vi "PXI UUT Control.vi"(1 "Enable Relays":bool, 2 "Reset IO":bool, 3 "error in (no error)":errorcluster {"code" format="%.0x"}, 4 "Enum":T2(ring), 5 "topology name":T1="2566/16-SPDT", 6 "resource name":refnum<k15>="PXI1Slot6") -> (0 "error out":errorcluster)   [LabVIEW 2014]
doc: "This VI conrtols the PXI communication streering relays.\nThe rountimes are:\n\nInit"
uses:
  <instrlib>/niSwitch/niswitch.llb/niSwitch Relay Action.ctl
  <instrlib>/niSwitch/niswitch.llb/niSwitch Topologies.ctl
panel:
  out "instrument handle out":refnum<k15>
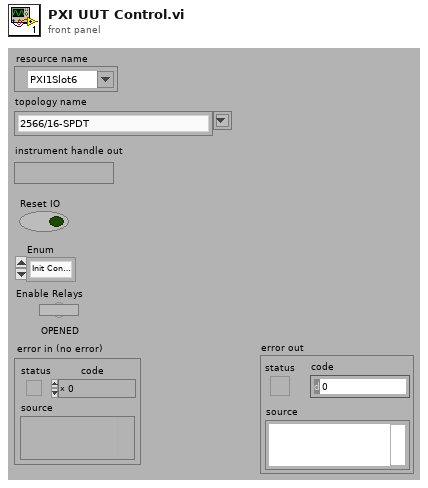
[diagram p1: front panel]
types:
  T1 = typedef "niSwitch Topologies.ctl" = string
  T2 = enum16{"Init Control Relays", "Secondary RS232", "Term Loopback", "CTS Isolate", "Synapse Loopback", "CST RTS Loopback", "Command Flash", "Auxillary RS232", "Battery Charge", "Remote Power", "Cordless Boot", "Auxillary Port", "DeInit Control Relays"}
  T3 = typedef "niSwitch Relay Action.ctl" = i32
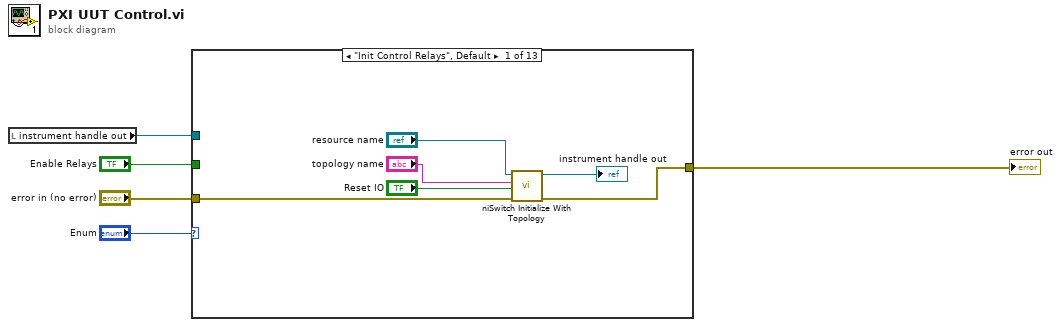
[diagram p0: block diagram]
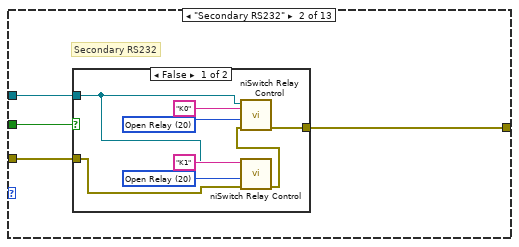
[diagram p2: hidden frame]
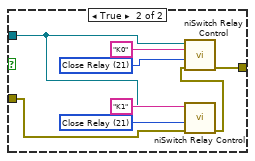
[diagram p3: hidden frame]
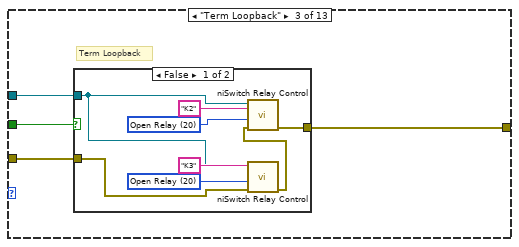
[diagram p4: hidden frame]
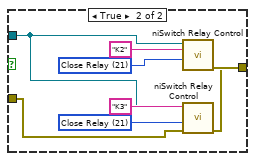
[diagram p5: hidden frame]
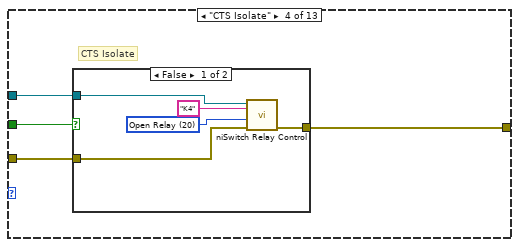
[diagram p6: hidden frame]
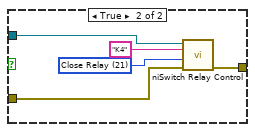
[diagram p7: hidden frame]
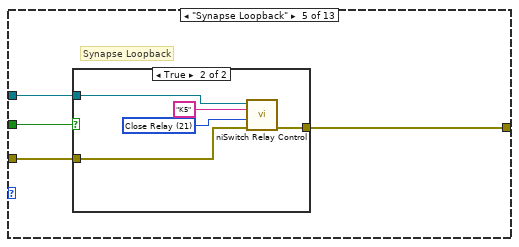
[diagram p8: hidden frame]
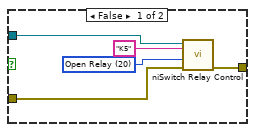
[diagram p9: hidden frame]
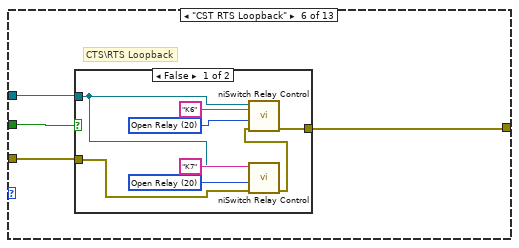
[diagram p10: hidden frame]
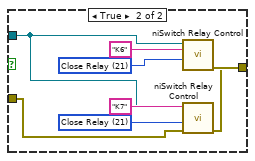
[diagram p11: hidden frame]
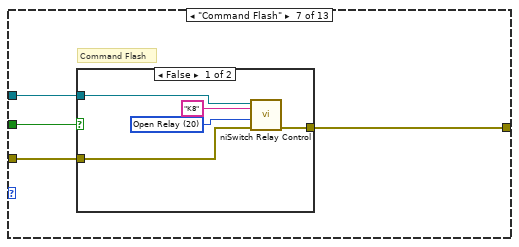
[diagram p12: hidden frame]
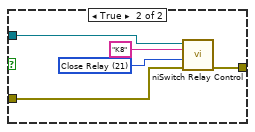
[diagram p13: hidden frame]
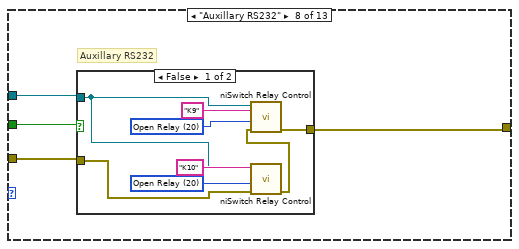
[diagram p14: hidden frame]
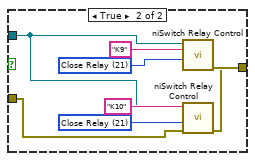
[diagram p15: hidden frame]
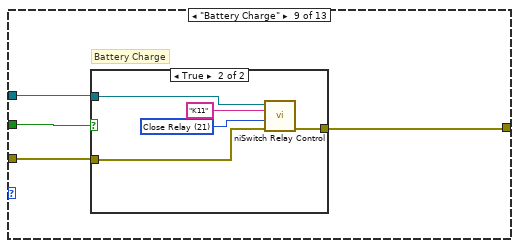
[diagram p16: hidden frame]
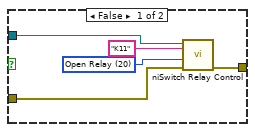
[diagram p17: hidden frame]
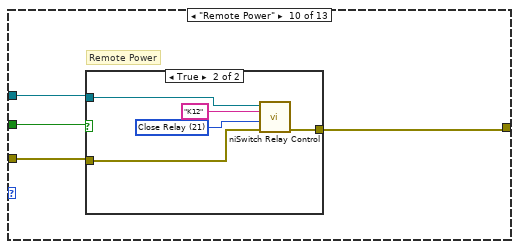
[diagram p18: hidden frame]
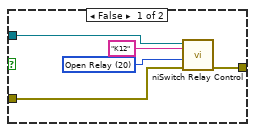
[diagram p19: hidden frame]
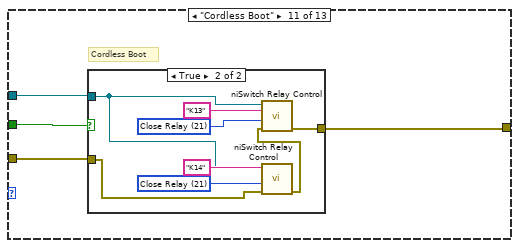
[diagram p20: hidden frame]
diagram:
  n1 = local read "instrument handle out"() -> (w4:refnum<k15>)
  n2 = case shown="\"Init Control Relays\", Default" "Enum" {
    tunnel: w4 -> [_ w15 w35 w55 w69 w83 w103 w117 w137 w151 w165 w184 w188]
    tunnel: [w11 w14 w32 w52 w66 w80 w100 w114 w134 w148 w162 w182 w185] -> w3
    tunnel: "Enable Relays" -> [_ w13 w34 w54 w68 w82 w102 w116 w136 w150 w164 _ w187]
    tunnel: "error in (no error)" -> [w10 w12 w33 w53 w67 w81 w101 w115 w135 w149 w163 w183 w186]
    frame "Init Control Relays", Default {
      n3 = call <instrlib>:"niSwitch Initialize With Topology.vi"("error in (no error)"=w10, "reset device (boolean value)"="Reset IO", "topology name"="topology name", "resource name"="resource name") -> ("error out"=w11:errorcluster, "instrument handle out"=→"instrument handle out":refnum<k15>)  [unwired: 6 in]
    }
    frame "Secondary RS232" {
      # "Secondary RS232"
      n4 = case shown="False" w13 {
        tunnel: [w21 w29] -> w14
        tunnel: w15 -> [w16 w24]
        tunnel: w12 -> [w17 w25]
        frame False {
          w20 = T3 20 items=["Open Relay"=20, "Close Relay"=21] ("relay action (Close Relay)")
          w23 = T3 20 items=["Open Relay"=20, "Close Relay"=21] ("relay action (Close Relay)")
          n5 = call <instrlib>:"niSwitch Relay Control.vi"("error in (no error)"=w17, "relay action (Close Relay)"=w20, "relay name"="K1", "instrument handle"=w16) -> ("error out"=w18:errorcluster)  [unwired: 6 in, 1 out]
          n6 = call <instrlib>:"niSwitch Relay Control.vi"("error in (no error)"=w18, "relay action (Close Relay)"=w23, "relay name"="K0", "instrument handle"=w16) -> ("error out"=w21:errorcluster)  [unwired: 6 in, 1 out]
        }
        frame True {
          w28 = T3 21 items=["Open Relay"=20, "Close Relay"=21] ("relay action (Close Relay)")
          w31 = T3 21 items=["Open Relay"=20, "Close Relay"=21] ("relay action (Close Relay)")
          n7 = call <instrlib>:"niSwitch Relay Control.vi"("error in (no error)"=w25, "relay action (Close Relay)"=w28, "relay name"="K1", "instrument handle"=w24) -> ("error out"=w26:errorcluster)  [unwired: 6 in, 1 out]
          n8 = call <instrlib>:"niSwitch Relay Control.vi"("error in (no error)"=w26, "relay action (Close Relay)"=w31, "relay name"="K0", "instrument handle"=w24) -> ("error out"=w29:errorcluster)  [unwired: 6 in, 1 out]
        }
      }
    }
    frame "Term Loopback" {
      # "Term Loopback"
      n9 = case shown="False" w34 {
        tunnel: w35 -> [w38 w46]
        tunnel: [w41 w49] -> w32
        tunnel: w33 -> [w36 w44]
        frame False {
          w40 = T3 20 items=["Open Relay"=20, "Close Relay"=21] ("relay action (Close Relay)")
          w43 = T3 20 items=["Open Relay"=20, "Close Relay"=21] ("relay action (Close Relay)")
          n10 = call <instrlib>:"niSwitch Relay Control.vi"("error in (no error)"=w36, "relay action (Close Relay)"=w40, "relay name"="K3", "instrument handle"=w38) -> ("error out"=w37:errorcluster)  [unwired: 6 in, 1 out]
          n11 = call <instrlib>:"niSwitch Relay Control.vi"("error in (no error)"=w37, "relay action (Close Relay)"=w43, "relay name"="K2", "instrument handle"=w38) -> ("error out"=w41:errorcluster)  [unwired: 6 in, 1 out]
        }
        frame True {
          w48 = T3 21 items=["Open Relay"=20, "Close Relay"=21] ("relay action (Close Relay)")
          w51 = T3 21 items=["Open Relay"=20, "Close Relay"=21] ("relay action (Close Relay)")
          n12 = call <instrlib>:"niSwitch Relay Control.vi"("error in (no error)"=w44, "relay action (Close Relay)"=w48, "relay name"="K3", "instrument handle"=w46) -> ("error out"=w45:errorcluster)  [unwired: 6 in, 1 out]
          n13 = call <instrlib>:"niSwitch Relay Control.vi"("error in (no error)"=w45, "relay action (Close Relay)"=w51, "relay name"="K2", "instrument handle"=w46) -> ("error out"=w49:errorcluster)  [unwired: 6 in, 1 out]
        }
      }
    }
    frame "CTS Isolate" {
      # "CTS Isolate"
      n14 = case shown="False" w54 {
        tunnel: w55 -> [w57 w62]
        tunnel: [w58 w63] -> w52
        tunnel: w53 -> [w56 w61]
        frame False {
          w60 = T3 20 items=["Open Relay"=20, "Close Relay"=21] ("relay action (Close Relay)")
          n15 = call <instrlib>:"niSwitch Relay Control.vi"("error in (no error)"=w56, "relay action (Close Relay)"=w60, "relay name"="K4", "instrument handle"=w57) -> ("error out"=w58:errorcluster)  [unwired: 6 in, 1 out]
        }
        frame True {
          w65 = T3 21 items=["Open Relay"=20, "Close Relay"=21] ("relay action (Close Relay)")
          n16 = call <instrlib>:"niSwitch Relay Control.vi"("error in (no error)"=w61, "relay action (Close Relay)"=w65, "relay name"="K4", "instrument handle"=w62) -> ("error out"=w63:errorcluster)  [unwired: 6 in, 1 out]
        }
      }
    }
    frame "Synapse Loopback" {
      # "Synapse Loopback"
      n17 = case shown="True" w68 {
        tunnel: w69 -> [w71 w76]
        tunnel: [w72 w77] -> w66
        tunnel: w67 -> [w70 w75]
        frame False {
          w74 = T3 20 items=["Open Relay"=20, "Close Relay"=21] ("relay action (Close Relay)")
          n18 = call <instrlib>:"niSwitch Relay Control.vi"("error in (no error)"=w70, "relay action (Close Relay)"=w74, "relay name"="K5", "instrument handle"=w71) -> ("error out"=w72:errorcluster)  [unwired: 6 in, 1 out]
        }
        frame True {
          w79 = T3 21 items=["Open Relay"=20, "Close Relay"=21] ("relay action (Close Relay)")
          n19 = call <instrlib>:"niSwitch Relay Control.vi"("error in (no error)"=w75, "relay action (Close Relay)"=w79, "relay name"="K5", "instrument handle"=w76) -> ("error out"=w77:errorcluster)  [unwired: 6 in, 1 out]
        }
      }
    }
    frame "CST RTS Loopback" {
      # "CTS\\RTS Loopback"
      n20 = case shown="False" w82 {
        tunnel: w83 -> [w86 w94]
        tunnel: [w89 w97] -> w80
        tunnel: w81 -> [w84 w92]
        frame False {
          w88 = T3 20 items=["Open Relay"=20, "Close Relay"=21] ("relay action (Close Relay)")
          w91 = T3 20 items=["Open Relay"=20, "Close Relay"=21] ("relay action (Close Relay)")
          n21 = call <instrlib>:"niSwitch Relay Control.vi"("error in (no error)"=w84, "relay action (Close Relay)"=w88, "relay name"="K7", "instrument handle"=w86) -> ("error out"=w85:errorcluster)  [unwired: 6 in, 1 out]
          n22 = call <instrlib>:"niSwitch Relay Control.vi"("error in (no error)"=w85, "relay action (Close Relay)"=w91, "relay name"="K6", "instrument handle"=w86) -> ("error out"=w89:errorcluster)  [unwired: 6 in, 1 out]
        }
        frame True {
          w96 = T3 21 items=["Open Relay"=20, "Close Relay"=21] ("relay action (Close Relay)")
          w99 = T3 21 items=["Open Relay"=20, "Close Relay"=21] ("relay action (Close Relay)")
          n23 = call <instrlib>:"niSwitch Relay Control.vi"("error in (no error)"=w92, "relay action (Close Relay)"=w96, "relay name"="K7", "instrument handle"=w94) -> ("error out"=w93:errorcluster)  [unwired: 6 in, 1 out]
          n24 = call <instrlib>:"niSwitch Relay Control.vi"("error in (no error)"=w93, "relay action (Close Relay)"=w99, "relay name"="K6", "instrument handle"=w94) -> ("error out"=w97:errorcluster)  [unwired: 6 in, 1 out]
        }
      }
    }
    frame "Command Flash" {
      # "Command Flash"
      n25 = case shown="False" w102 {
        tunnel: w103 -> [w105 w110]
        tunnel: [w106 w111] -> w100
        tunnel: w101 -> [w104 w109]
        frame False {
          w108 = T3 20 items=["Open Relay"=20, "Close Relay"=21] ("relay action (Close Relay)")
          n26 = call <instrlib>:"niSwitch Relay Control.vi"("error in (no error)"=w104, "relay action (Close Relay)"=w108, "relay name"="K8", "instrument handle"=w105) -> ("error out"=w106:errorcluster)  [unwired: 6 in, 1 out]
        }
        frame True {
          w113 = T3 21 items=["Open Relay"=20, "Close Relay"=21] ("relay action (Close Relay)")
          n27 = call <instrlib>:"niSwitch Relay Control.vi"("error in (no error)"=w109, "relay action (Close Relay)"=w113, "relay name"="K8", "instrument handle"=w110) -> ("error out"=w111:errorcluster)  [unwired: 6 in, 1 out]
        }
      }
    }
    frame "Auxillary RS232" {
      # "Auxillary RS232"
      n28 = case shown="False" w116 {
        tunnel: w117 -> [w120 w128]
        tunnel: [w123 w131] -> w114
        tunnel: w115 -> [w118 w126]
        frame False {
          w122 = T3 20 items=["Open Relay"=20, "Close Relay"=21] ("relay action (Close Relay)")
          w125 = T3 20 items=["Open Relay"=20, "Close Relay"=21] ("relay action (Close Relay)")
          n29 = call <instrlib>:"niSwitch Relay Control.vi"("error in (no error)"=w118, "relay action (Close Relay)"=w122, "relay name"="K10", "instrument handle"=w120) -> ("error out"=w119:errorcluster)  [unwired: 6 in, 1 out]
          n30 = call <instrlib>:"niSwitch Relay Control.vi"("error in (no error)"=w119, "relay action (Close Relay)"=w125, "relay name"="K9", "instrument handle"=w120) -> ("error out"=w123:errorcluster)  [unwired: 6 in, 1 out]
        }
        frame True {
          w130 = T3 21 items=["Open Relay"=20, "Close Relay"=21] ("relay action (Close Relay)")
          w133 = T3 21 items=["Open Relay"=20, "Close Relay"=21] ("relay action (Close Relay)")
          n31 = call <instrlib>:"niSwitch Relay Control.vi"("error in (no error)"=w126, "relay action (Close Relay)"=w130, "relay name"="K10", "instrument handle"=w128) -> ("error out"=w127:errorcluster)  [unwired: 6 in, 1 out]
          n32 = call <instrlib>:"niSwitch Relay Control.vi"("error in (no error)"=w127, "relay action (Close Relay)"=w133, "relay name"="K9", "instrument handle"=w128) -> ("error out"=w131:errorcluster)  [unwired: 6 in, 1 out]
        }
      }
    }
    frame "Battery Charge" {
      # "Battery Charge"
      n33 = case shown="True" w136 {
        tunnel: w137 -> [w139 w144]
        tunnel: [w140 w145] -> w134
        tunnel: w135 -> [w138 w143]
        frame False {
          w142 = T3 20 items=["Open Relay"=20, "Close Relay"=21] ("relay action (Close Relay)")
          n34 = call <instrlib>:"niSwitch Relay Control.vi"("error in (no error)"=w138, "relay action (Close Relay)"=w142, "relay name"="K11", "instrument handle"=w139) -> ("error out"=w140:errorcluster)  [unwired: 6 in, 1 out]
        }
        frame True {
          w147 = T3 21 items=["Open Relay"=20, "Close Relay"=21] ("relay action (Close Relay)")
          n35 = call <instrlib>:"niSwitch Relay Control.vi"("error in (no error)"=w143, "relay action (Close Relay)"=w147, "relay name"="K11", "instrument handle"=w144) -> ("error out"=w145:errorcluster)  [unwired: 6 in, 1 out]
        }
      }
    }
    frame "Remote Power" {
      # "Remote Power"
      n36 = case shown="True" w150 {
        tunnel: w151 -> [w153 w158]
        tunnel: [w154 w159] -> w148
        tunnel: w149 -> [w152 w157]
        frame False {
          w156 = T3 20 items=["Open Relay"=20, "Close Relay"=21] ("relay action (Close Relay)")
          n37 = call <instrlib>:"niSwitch Relay Control.vi"("error in (no error)"=w152, "relay action (Close Relay)"=w156, "relay name"="K12", "instrument handle"=w153) -> ("error out"=w154:errorcluster)  [unwired: 6 in, 1 out]
        }
        frame True {
          w161 = T3 21 items=["Open Relay"=20, "Close Relay"=21] ("relay action (Close Relay)")
          n38 = call <instrlib>:"niSwitch Relay Control.vi"("error in (no error)"=w157, "relay action (Close Relay)"=w161, "relay name"="K12", "instrument handle"=w158) -> ("error out"=w159:errorcluster)  [unwired: 6 in, 1 out]
        }
      }
    }
    frame "Cordless Boot" {
      # "Cordless Boot"
      n39 = case shown="True" w164 {
        tunnel: w165 -> [w168 w176]
        tunnel: [w171 w179] -> w162
        tunnel: w163 -> [w166 w174]
        frame False {
          w170 = T3 20 items=["Open Relay"=20, "Close Relay"=21] ("relay action (Close Relay)")
          w173 = T3 20 items=["Open Relay"=20, "Close Relay"=21] ("relay action (Close Relay)")
          n40 = call <instrlib>:"niSwitch Relay Control.vi"("error in (no error)"=w166, "relay action (Close Relay)"=w170, "relay name"="K14", "instrument handle"=w168) -> ("error out"=w167:errorcluster)  [unwired: 6 in, 1 out]
          n41 = call <instrlib>:"niSwitch Relay Control.vi"("error in (no error)"=w167, "relay action (Close Relay)"=w173, "relay name"="K13", "instrument handle"=w168) -> ("error out"=w171:errorcluster)  [unwired: 6 in, 1 out]
        }
        frame True {
          w178 = T3 21 items=["Open Relay"=20, "Close Relay"=21] ("relay action (Close Relay)")
          w181 = T3 21 items=["Open Relay"=20, "Close Relay"=21] ("relay action (Close Relay)")
          n42 = call <instrlib>:"niSwitch Relay Control.vi"("error in (no error)"=w174, "relay action (Close Relay)"=w178, "relay name"="K14", "instrument handle"=w176) -> ("error out"=w175:errorcluster)  [unwired: 6 in, 1 out]
          n43 = call <instrlib>:"niSwitch Relay Control.vi"("error in (no error)"=w175, "relay action (Close Relay)"=w181, "relay name"="K13", "instrument handle"=w176) -> ("error out"=w179:errorcluster)  [unwired: 6 in, 1 out]
        }
      }
    }
    frame "DeInit Control Relays" {
      n44 = call <instrlib>:"niSwitch Close.vi"("error in (no error)"=w183, "instrument handle"=w184) -> ("error out"=w182:errorcluster)  [unwired: 9 in]
    }
    frame "Auxillary Port" {
      # "Auxillary Power"
      n45 = case shown="True" w187 {
        tunnel: w188 -> [w190 w195]
        tunnel: [w191 w196] -> w185
        tunnel: w186 -> [w189 w194]
        frame False {
          w193 = T3 20 items=["Open Relay"=20, "Close Relay"=21] ("relay action (Close Relay)")
          n46 = call <instrlib>:"niSwitch Relay Control.vi"("error in (no error)"=w189, "relay action (Close Relay)"=w193, "relay name"="K15", "instrument handle"=w190) -> ("error out"=w191:errorcluster)  [unwired: 6 in, 1 out]
        }
        frame True {
          w198 = T3 21 items=["Open Relay"=20, "Close Relay"=21] ("relay action (Close Relay)")
          n47 = call <instrlib>:"niSwitch Relay Control.vi"("error in (no error)"=w194, "relay action (Close Relay)"=w198, "relay name"="K15", "instrument handle"=w195) -> ("error out"=w196:errorcluster)  [unwired: 6 in, 1 out]
        }
      }
    }
  }
  "error out" <- w3
